vi "OBJ_MAIN_history_arrays.vi"(5 "item_names_in":string[][](array[string]), 7 "statuses_in":T3[](array[typedef]), 9 "tests_to_remember":i32, 11 "output cluster":T1) -> (2 "statuses_out":T3[](array[typedef]), 3 "item_names_out":string[][](array[string]))   [LabVIEW 2019]
uses:
  OBJ_measurement_status.ctl
  FGV/OBJ_records_display/OBJ_all_info.ctl
  OBJ_header_data_display.ctl
  FGV/OBJ_records_display/OBJ_references.ctl
panel:
  # "GEAR INFO SUMMARY"
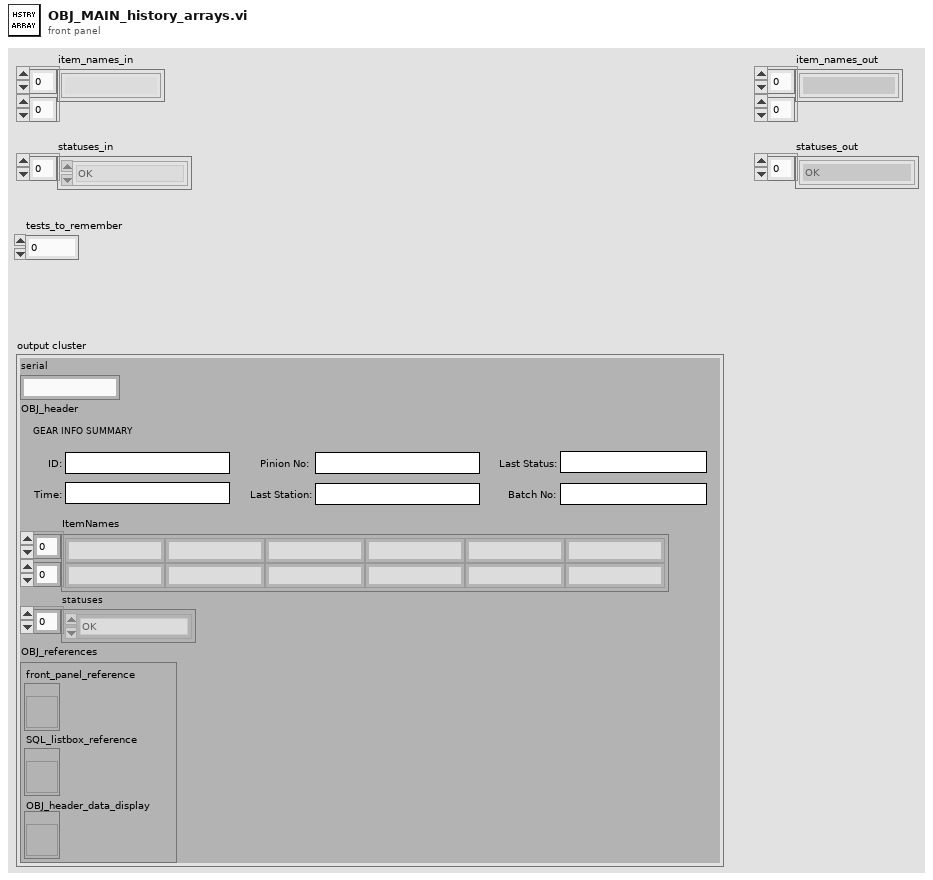
[diagram p1: front panel]
types:
  T1 = typedef "OBJ_all_info.ctl" = cluster{"serial":string, "OBJ_header":T2, "ItemNames":string[][], "statuses":T3[], "OBJ_references":T4}
  T2 = typedef "OBJ_header_data_display.ctl" = cluster{"ID":string, "creation_time":string, "last_station":string, "last_status":string, "pinion_serial":string, "batch_code":string}
  T3 = typedef "OBJ_measurement_status.ctl" = enum16{"OK", "NOK"}
  T4 = typedef "OBJ_references.ctl" = cluster{"front_panel_reference":refnum<vi>, "SQL_listbox_reference":refnum<vi>, "OBJ_header_data_display":refnum<vi>}
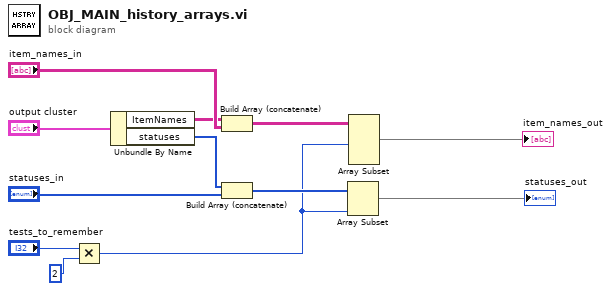
[diagram p0: block diagram]
diagram:
  n1 = Multiply(x="tests_to_remember", y=2) -> (x*y=w7:i32)
  n2 = Unbundle By Name("output cluster") -> ("ItemNames"=w3:string[][], "statuses"=w2:T3[])
  n3 = Build Array (concatenate)(w3, "item_names_in") -> (w11:string[][])
  n4 = Build Array (concatenate)(w2, "statuses_in") -> (w8:T3[])
  n5 = Array Subset(array=w8, length=w7) -> (→"statuses_out":T3[])  [unwired: 1 in]
  n6 = Array Subset(array=w11, length (row)=w7) -> (→"item_names_out":string[][])  [unwired: 3 in]
